vi "Destroy PrimeTimer Q.vi"(8 "error in (no error)":errorcluster) -> (0 "error out":errorcluster, 3 "Final Data":variant[](array[variant]))   [LabVIEW 2022 SP3, in "DAQ.lvclass"]
doc: "Developed by Kevin Thompson\nThompson Engineering, LLC\nkevin@thompsonengineering.net"
uses:
  TD DaqLoopTime DataQ--ref.ctl
  GBL DataQ Refs.vi
  DAQ.lvclass
  DAQ.lvclass/DAQ.ctl
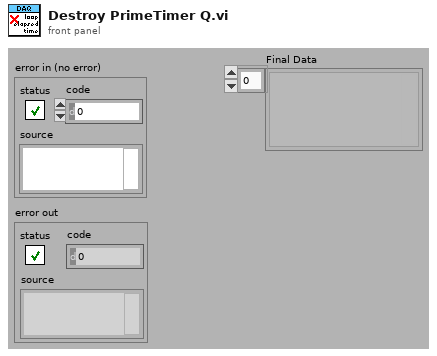
[diagram p1: front panel]
types:
  T1 = typedef "DAQ.lvclass/TD DaqLoopTime DataQ--ref.ctl" = refnum<queue>
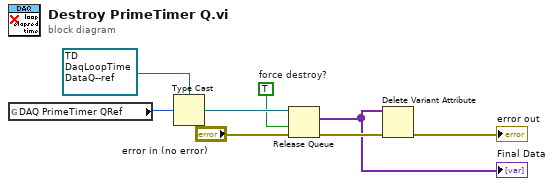
[diagram p0: block diagram]
diagram:
  w4 = TRUE  # force destroy?
  n1 = global read "GBL DataQ Refs.vi" "DAQ PrimeTimer QRef"() -> (w5:u32)
  n2 = Type Cast(type=T1 refnum ("DaqData ElapsedTimeRef"), x=w5) -> (*(type *) &x=w7:T1)
  n3 = Release Queue(queue=w7, force destroy? (F)=w4, error in (no error)="error in (no error)") -> (remaining elements=w2:variant[], error out=w3:errorcluster)  [unwired: 1 out]
  "Final Data" <- w2
  n4 = Delete Variant Attribute(4:w3, 7:w2) -> (0:→"error out":errorcluster)  [unwired: 1 in, 2 out]
